vi "sub_calc-repulsive_potential.vi"(9 "rr":dbl, 10 "obstacles":cluster{"x":dbl, "y":dbl}[](array[cluster]), 11 "xy pt":cluster{"x":dbl, "y":dbl}) -> (3 "return":dbl)   [LabVIEW 2019]
uses:
  Ctrl/cmd_common.ctl
panel:
  out "dmin":dbl=-1.0 format="%#_13g"
  out "minid":i32=-1
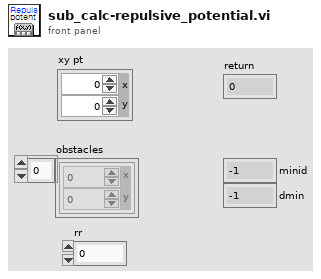
[diagram p1: front panel]
types:
  T1 = typedef "cmd_common.ctl" = enum16{"read", "write"}
  T2 = cluster{"KP":dbl, "ETA":dbl, "AREA_WIDTH":dbl, "Osc_Det_Len":u32}
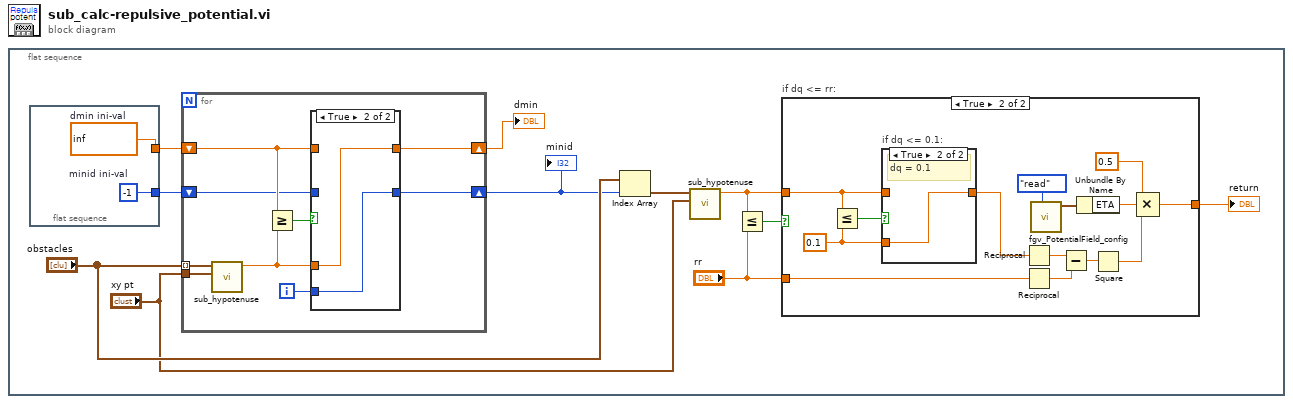
[diagram p0: block diagram]
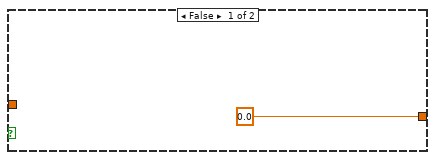
[diagram p2: hidden frame]
diagram:
  n1 = flat-sequence {
    frame #0 {
      n2 = flat-sequence {
        tunnel: [w30] -> w11
        tunnel: [w29] -> w10
        frame #0 {
          w29 = -1  # minid ini-val
          w30 = inf  # dmin ini-val
        }
      }
      n3 = for {
        tunnel: "obstacles" -> [w39] mode=indexing
        tunnel: "xy pt" -> [w38]
        shift-right: [w36] -> w9
        shift-left: w11 -> [w34]
        shift-right: [w33] -> w7
        shift-left: w10 -> [w32]
        i -> [w31]
        n4 = call "sub_hypotenuse.vi"("x2y2"=w38, "x1y1"=w39) -> ("length"=w35:dbl)  [unwired: 9 in]
        n5 = Greater Or Equal?(x=w34, y=w35) -> (x >= y?=w37:bool)
        n6 = case shown="True" w37 {
          tunnel: [w41 w43] -> w36
          tunnel: w35 -> [_ w43]
          tunnel: w34 -> [w41 _]
          tunnel: [w40 w42] -> w33
          tunnel: w32 -> [w40 _]
          tunnel: w31 -> [_ w42]
          frame False {
          }
          frame True {
          }
        }
      }
      "dmin" <- w9
      "minid" <- w7
      n7 = Index Array(array="obstacles", index=w7) -> (element=w5:cluster{"x":dbl, "y":dbl})
      n8 = call "sub_hypotenuse.vi"("x2y2"="xy pt", "x1y1"=w5) -> ("length"=w3:dbl)  [unwired: 9 in]
      n9 = Less Or Equal?(x=w3, y="rr") -> (x <= y?=w4:bool)
      n10 = case "if dq <= rr:" shown="True" w4 {
        tunnel: w3 -> [_ w20]
        tunnel: [0.0 ("length") w14] -> w1
        tunnel: "rr" -> [_ w19]
        frame False {
          # "return non xrto"
        }
        frame True {
          w25 = 0.1 ("y")
          n11 = Less Or Equal?(x=w20, y=w25) -> (x <= y?=w26:bool)
          n12 = case "if dq <= 0.1:" shown="True" w26 {
            tunnel: [w27 w28] -> w13
            tunnel: w20 -> [w27 _]
            tunnel: w25 -> [_ w28]
            frame False {
            }
            frame True {
              # "dq = 0.1"
            }
          }
          n13 = Reciprocal(x=w13) -> (1/x=w18:dbl)
          n14 = Reciprocal(x=w19) -> (1/x=w17:dbl)
          n15 = call "fgv_PotentialField_config.vi"("cmd"=cmd_common."read") -> ("pf-val out"=w23:T2)  [unwired: 10 in]
          n16 = Subtract(x=w18, y=w17) -> (x-y=w16:dbl)
          n17 = Unbundle By Name(w23) -> ("ETA"=w22:dbl)
          n18 = Square(x=w16) -> (x^2=w15:dbl)
          n19 = Compound Arithmetic op=MULTIPLY(0.5 ("value"), w22, w15) -> (w14:dbl)
        }
      }
      "return" <- w1
    }
  }
